vi "Nyq&Log.vi"() -> ()   [LabVIEW 2017]
uses:
  <vilib>/Instr/_visa.llb/VISA Configure Serial Port (Instr).vi
panel:
  in  "stop logging":bool
  out "Imaginary":dbl(graph)
  out "Real":dbl(graph)
  out "imaginar":string
  out "real":string
  out "return count 2":u32
  out "read buffer 6":string
  out "read buffer 7":string
  out "read buffer 5":string
  out "read buffer 4":string
  out "logging freq":string
  in  "logging Freq":i32
  out "Nyquest plot":cluster{dbl[], dbl[]}(graph)
  out "read buffer 2":string
  out "read buffer 3":string
  out "read buffer":string
  out "return count":u32
  out "Sweep Parameter":string
  out "Imaginary":string
  out "Real":string
  in  "No. of steps":i32
  in  "Freq Step":dbl
  in  "Start Freq":dbl
  in  "stop":bool
  in  "Radio Buttons":enum32{"0", "1", "2"}(radio)
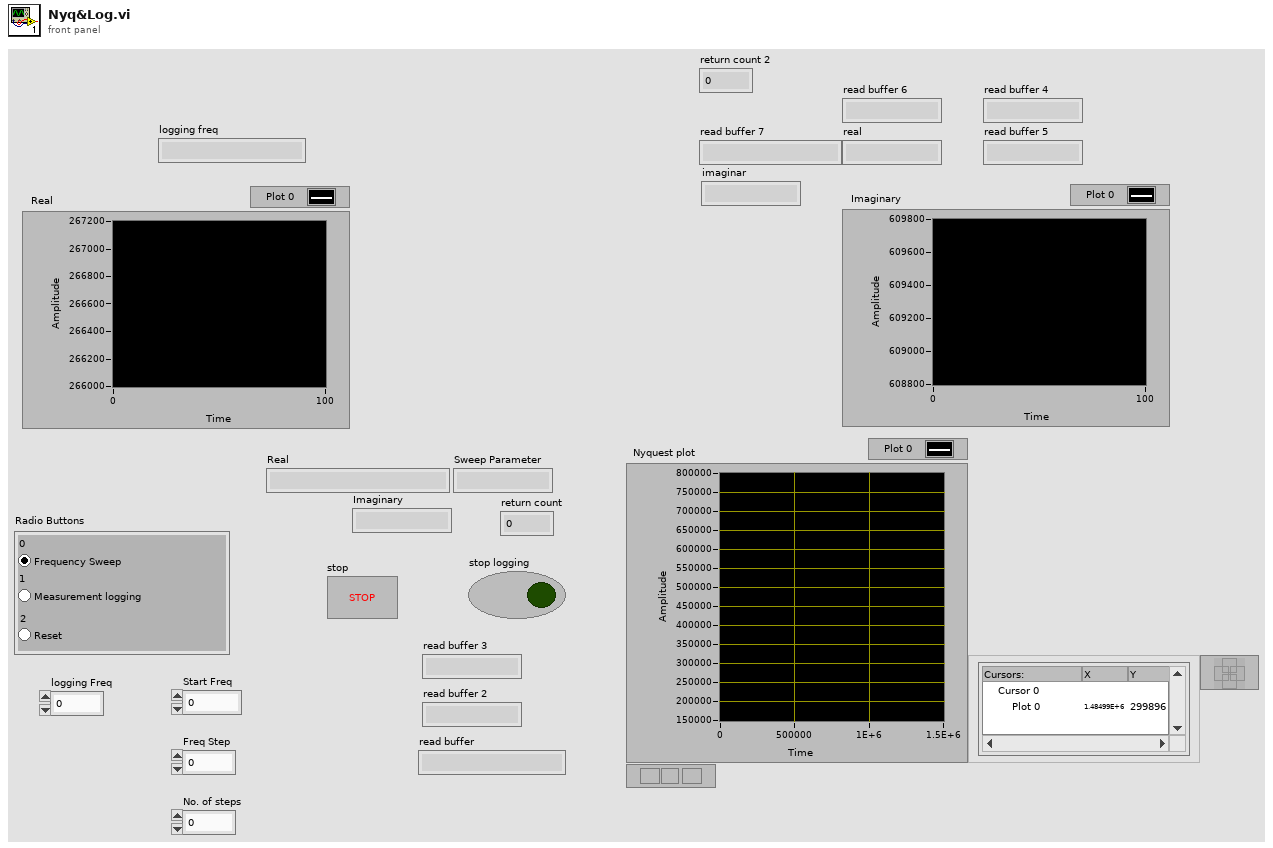
[diagram p1: front panel]
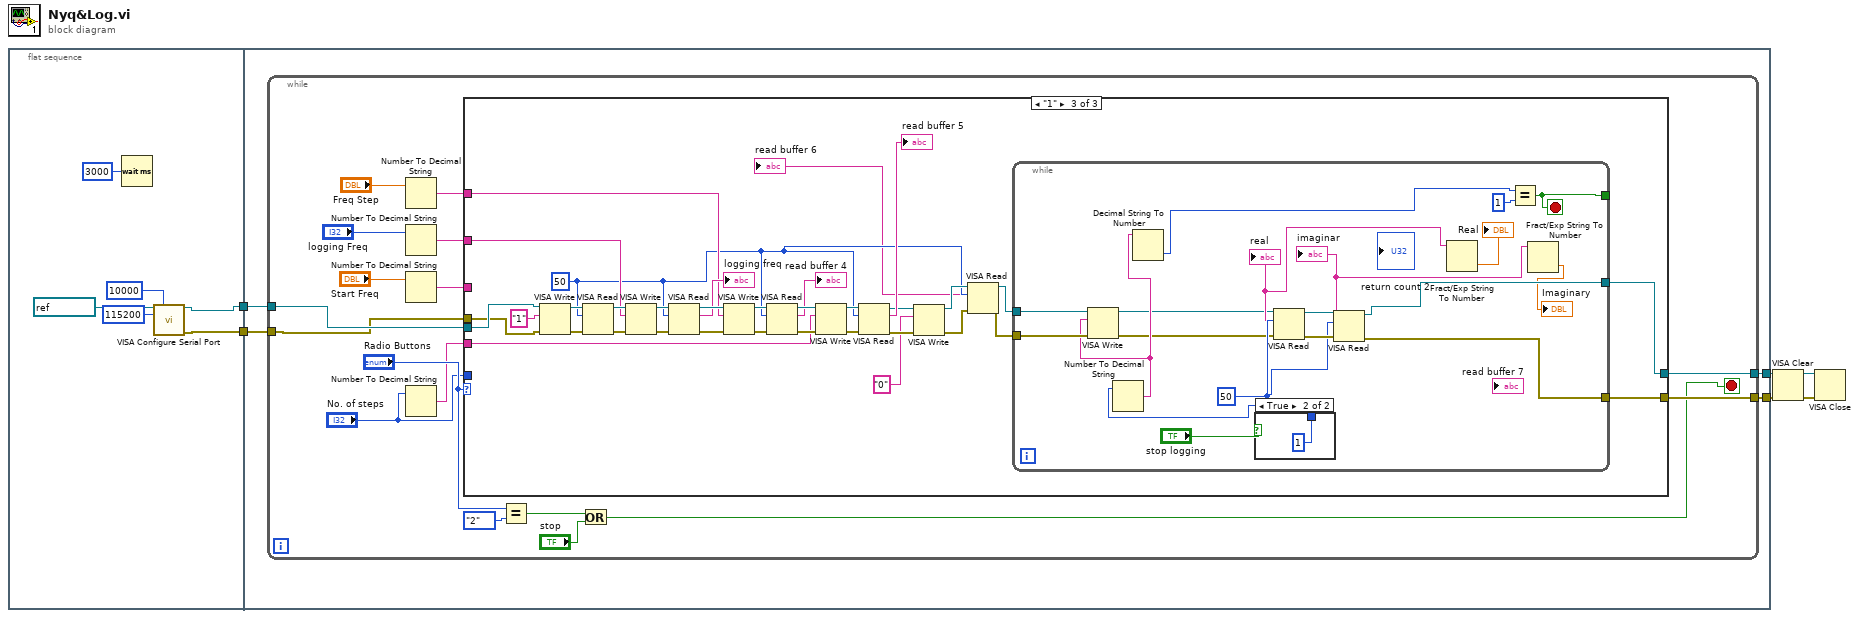
[diagram p0: block diagram]
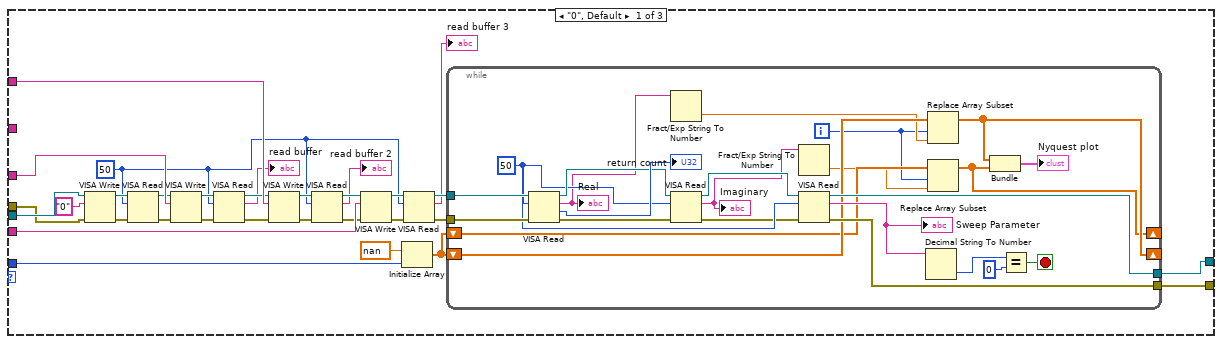
[diagram p2: hidden frame]
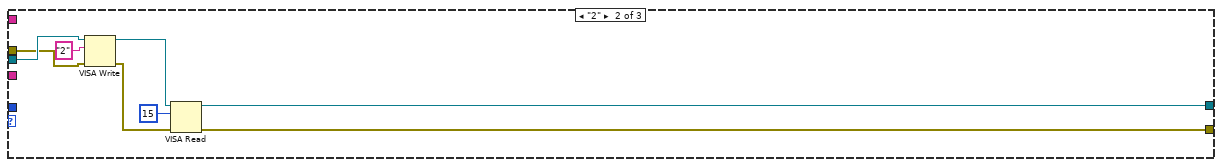
[diagram p3: hidden frame]
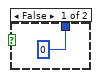
[diagram p4: hidden frame]
diagram:
  n1 = flat-sequence {
    tunnel: [w10] -> w2
    tunnel: [w9] -> w1
    tunnel: [w14] -> w4
    tunnel: [w13] -> w3
    tunnel: w2 -> [w16]
    tunnel: w1 -> [w15]
    frame #0 {
      n2 = Wait (ms)(milliseconds to wait=u32 3000) -> ()  [unwired: 1 out]
      n3 = call-poly "VISA Configure Serial Port"("VISA resource name"=refnum<visa-resource-name> "COM4", "timeout (10sec)"=u32 10000, "baud rate (9600)"=u32 115200) -> ("VISA resource name out"=w10:refnum<visa-resource-name>, "error out"=w9:errorcluster)  [unwired: 11 in]
    }
    frame #1 {
      n4 = while {
        tunnel: w16 -> [w19]
        tunnel: w15 -> [w18]
        tunnel: [w29] -> w13
        tunnel: [w28] -> w14
        stop <- w17 stop-if-true
        n5 = Number To Decimal String(number="Freq Step") -> (decimal integer string=w23:string)  [unwired: 1 in]
        n6 = Number To Decimal String(number="logging Freq") -> (decimal integer string=w20:string)  [unwired: 1 in]
        n7 = Number To Decimal String(number="Start Freq") -> (decimal integer string=w25:string)  [unwired: 1 in]
        n8 = Number To Decimal String(number="No. of steps") -> (decimal integer string=w27:string)  [unwired: 1 in]
        n9 = case shown="\"1\"" "Radio Buttons" {
          tunnel: [w61 w96 w102] -> w28
          tunnel: [w60 w95 w101] -> w29
          tunnel: w25 -> [w64 _ _]
          tunnel: w23 -> [w63 _ w114]
          tunnel: w27 -> [w62 _ w113]
          tunnel: "No. of steps" -> [w37 _ _]
          tunnel: w20 -> [_ _ w112]
          tunnel: w19 -> [w35 w90 w98]
          tunnel: w18 -> [w34 w89 w97]
          frame "0", Default {
            w42 = u32 50 ("byte count")
            n10 = VISA Write(VISA resource name=w35, write buffer="0", error in (no error)=w34) -> (VISA resource name out=w57:refnum<visa-resource-name>, error out=w59:errorcluster)  [unwired: 1 out]
            n11 = VISA Read(VISA resource name=w57, byte count=w42, error in (no error)=w59) -> (VISA resource name out=w56:refnum<visa-resource-name>, error out=w55:errorcluster)  [unwired: 2 out]
            n12 = VISA Write(VISA resource name=w56, write buffer=w64, error in (no error)=w55) -> (VISA resource name out=w54:refnum<visa-resource-name>, error out=w53:errorcluster)  [unwired: 1 out]
            n13 = VISA Read(VISA resource name=w54, byte count=w42, error in (no error)=w53) -> (VISA resource name out=w52:refnum<visa-resource-name>, read buffer=→"read buffer":string, error out=w51:errorcluster)  [unwired: 1 out]
            n14 = VISA Write(VISA resource name=w52, write buffer=w63, error in (no error)=w51) -> (VISA resource name out=w50:refnum<visa-resource-name>, error out=w49:errorcluster)  [unwired: 1 out]
            n15 = VISA Read(VISA resource name=w50, byte count=w42, error in (no error)=w49) -> (VISA resource name out=w48:refnum<visa-resource-name>, read buffer=→"read buffer 2":string, error out=w47:errorcluster)  [unwired: 1 out]
            n16 = VISA Write(VISA resource name=w48, write buffer=w62, error in (no error)=w47) -> (VISA resource name out=w46:refnum<visa-resource-name>, error out=w45:errorcluster)  [unwired: 1 out]
            n17 = Initialize Array(nan ("element"), w37) -> (w36:dbl[])
            n18 = VISA Read(VISA resource name=w46, byte count=w42, error in (no error)=w45) -> (VISA resource name out=w44:refnum<visa-resource-name>, read buffer=→"read buffer 3":string, error out=w43:errorcluster)  [unwired: 1 out]
            n19 = while {
              tunnel: w44 -> [w88]
              tunnel: w43 -> [w87]
              tunnel: [w77] -> w61
              tunnel: [w76] -> w60
              shift-right: [w70] -> _
              shift-left: w36 -> [w72]
              shift-right: [w66] -> _
              shift-left: w36 -> [w69]
              i -> [w67]
              stop <- w84 stop-if-true
              w80 = u32 50 ("byte count")
              n20 = VISA Read(VISA resource name=w88, byte count=w80, error in (no error)=w87) -> (VISA resource name out=w82:refnum<visa-resource-name>, read buffer=w74:string, return count=→"return count":u32, error out=w81:errorcluster)
              "Real" <- w74
              n21 = Fract/Exp String To Number(string=w74) -> (number=w71:dbl)  [unwired: 3 in, 1 out]
              n22 = VISA Read(VISA resource name=w82, byte count=w80, error in (no error)=w81) -> (VISA resource name out=w79:refnum<visa-resource-name>, read buffer=w73:string, error out=w78:errorcluster)  [unwired: 1 out]
              "Imaginary" <- w73
              n23 = Fract/Exp String To Number(string=w73) -> (number=w68:dbl)  [unwired: 3 in, 1 out]
              n24 = VISA Read(VISA resource name=w79, byte count=w80, error in (no error)=w78) -> (VISA resource name out=w77:refnum<visa-resource-name>, read buffer=w75:string, error out=w76:errorcluster)  [unwired: 1 out]
              "Sweep Parameter" <- w75
              n25 = Decimal String To Number(string=w75) -> (number=w86:i32)  [unwired: 2 in, 1 out]
              n26 = Replace Array Subset(array=w72, new element=w71, index=w67) -> (w70:dbl[])
              n27 = Replace Array Subset(array=w69, new element=w68, index=w67) -> (w66:dbl[])
              n28 = Bundle(w70, w66) -> (→"Nyquest plot":cluster{dbl[], dbl[]})  [unwired: 1 in]
              n29 = Equal?(x=w86, y=0) -> (x = y?=w84:bool)
            }
          }
          frame "2" {
            n30 = VISA Write(VISA resource name=w90, write buffer="2", error in (no error)=w89) -> (VISA resource name out=w93:refnum<visa-resource-name>, error out=w92:errorcluster)  [unwired: 1 out]
            n31 = VISA Read(VISA resource name=w93, byte count=u32 15, error in (no error)=w92) -> (VISA resource name out=w96:refnum<visa-resource-name>, error out=w95:errorcluster)  [unwired: 2 out]
          }
          frame "1" {
            w104 = u32 50 ("byte count")
            n32 = VISA Write(VISA resource name=w98, write buffer="1", error in (no error)=w97) -> (VISA resource name out=w128:refnum<visa-resource-name>, error out=w130:errorcluster)  [unwired: 1 out]
            n33 = VISA Read(VISA resource name=w128, byte count=w104, error in (no error)=w130) -> (VISA resource name out=w127:refnum<visa-resource-name>, error out=w126:errorcluster)  [unwired: 2 out]
            n34 = VISA Write(VISA resource name=w127, write buffer=w112, error in (no error)=w126) -> (VISA resource name out=w125:refnum<visa-resource-name>, error out=w124:errorcluster)  [unwired: 1 out]
            n35 = VISA Read(VISA resource name=w125, byte count=w104, error in (no error)=w124) -> (VISA resource name out=w123:refnum<visa-resource-name>, read buffer=→"logging freq":string, error out=w122:errorcluster)  [unwired: 1 out]
            n36 = VISA Write(VISA resource name=w123, write buffer=w114, error in (no error)=w122) -> (VISA resource name out=w121:refnum<visa-resource-name>, error out=w120:errorcluster)  [unwired: 1 out]
            n37 = VISA Read(VISA resource name=w121, byte count=w104, error in (no error)=w120) -> (VISA resource name out=w119:refnum<visa-resource-name>, read buffer=→"read buffer 4":string, error out=w118:errorcluster)  [unwired: 1 out]
            n38 = VISA Write(VISA resource name=w119, write buffer=w113, error in (no error)=w118) -> (VISA resource name out=w117:refnum<visa-resource-name>, error out=w116:errorcluster)  [unwired: 1 out]
            n39 = VISA Read(VISA resource name=w117, byte count=w104, error in (no error)=w116) -> (VISA resource name out=w109:refnum<visa-resource-name>, read buffer=→"read buffer 5":string, error out=w108:errorcluster)  [unwired: 1 out]
            n40 = VISA Write(VISA resource name=w109, write buffer="0", error in (no error)=w108) -> (VISA resource name out=w106:refnum<visa-resource-name>, error out=w105:errorcluster)  [unwired: 1 out]
            n41 = VISA Read(VISA resource name=w106, byte count=w104, error in (no error)=w105) -> (VISA resource name out=w100:refnum<visa-resource-name>, read buffer=→"read buffer 6":string, error out=w99:errorcluster)  [unwired: 1 out]
            n42 = while {
              tunnel: [w148] -> _
              tunnel: w100 -> [w146]
              tunnel: w99 -> [w145]
              tunnel: [w140] -> w102
              tunnel: [w139] -> w101
              stop <- w148 stop-if-true
              w141 = u32 50 ("byte count")
              n43 = case shown="True" "stop logging" {
                tunnel: [0 1] -> w131
                frame False {
                }
                frame True {
                }
              }
              n44 = Number To Decimal String(number=w131) -> (decimal integer string=w144:string)  [unwired: 1 in]
              n45 = VISA Write(VISA resource name=w146, write buffer=w144, error in (no error)=w145) -> (VISA resource name out=w134:refnum<visa-resource-name>, error out=w133:errorcluster)  [unwired: 1 out]
              n46 = Decimal String To Number(string=w144) -> (number=w147:i32)  [unwired: 2 in, 1 out]
              n47 = VISA Read(VISA resource name=w134, byte count=w141, error in (no error)=w133) -> (VISA resource name out=w143:refnum<visa-resource-name>, read buffer=w138:string, error out=w142:errorcluster)  [unwired: 1 out]
              "real" <- w138
              n48 = VISA Read(VISA resource name=w143, byte count=w141, error in (no error)=w142) -> (VISA resource name out=w140:refnum<visa-resource-name>, read buffer=w137:string, error out=w139:errorcluster)  [unwired: 1 out]
              "imaginar" <- w137
              n49 = Fract/Exp String To Number(string=w138) -> (number=→"Real":dbl)  [unwired: 3 in, 1 out]
              n50 = Equal?(x=w147, y=1) -> (x = y?=w148:bool)
              n51 = Fract/Exp String To Number(string=w137) -> (number=→"Imaginary":dbl)  [unwired: 3 in, 1 out]
            }
          }
        }
        n52 = Equal?(x="Radio Buttons", y=enum32{"0", "1", "2"}."2") -> (x = y?=w32:bool)
        n53 = Or(x=w32, y="stop") -> (x .or. y?=w17:bool)
      }
    }
  }
  n54 = VISA Clear(VISA resource name=w4, error in (no error)=w3) -> (VISA resource name out=w6:refnum<visa-resource-name>, error out=w5:errorcluster)
  n55 = VISA Close(VISA resource name=w6, error in (no error)=w5) -> ()  [unwired: 1 out]
